vi "5.10 Fuzzy Average Function.vi"(1 "Input Control Certainty Array":dbl[][](array[numeric])) -> (0 "Output Control Value":dbl)   [LabVIEW 2011]
panel:
  out "Certainty Eta":dbl
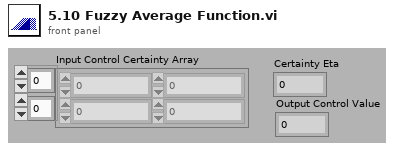
[diagram p1: front panel]
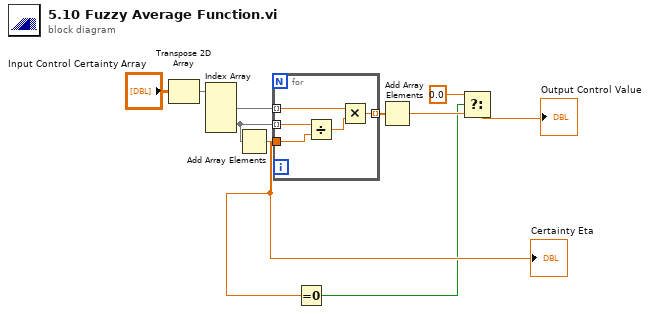
[diagram p0: block diagram]
diagram:
  n1 = Transpose 2D Array(2D array="Input Control Certainty Array") -> (transposed array=w9:dbl[][])
  n2 = Index Array(array=w9) -> (element #1=w8:dbl[], element #2=w7:dbl[])  [unwired: 4 in]
  n3 = Add Array Elements(numeric array=w7) -> (sum=w4:dbl)
  "Certainty Eta" <- w4
  n4 = for {
    tunnel: w8 -> [w12] mode=indexing
    tunnel: w7 -> [w15] mode=indexing
    tunnel: w4 -> [w14]
    tunnel: [w11] -> w6 mode=indexing
    n5 = Divide(x=w15, y=w14) -> (x/y=w13:dbl)
    n6 = Multiply(x=w12, y=w13) -> (x*y=w11:dbl)
  }
  n7 = Equal To 0?(x=w4) -> (x = 0?=w2:bool)
  n8 = Add Array Elements(numeric array=w6) -> (sum=w5:dbl)
  n9 = Select(t=0.0, s=w2, f=w5) -> (s? t:f=→"Output Control Value":dbl)
